vi "Calculate_Release_Flowrates.vi"(3 "Ch names":string[](array[string]), 4 "Units":enum16{"Q l/min", "M_dot Kg/min"}(ring), 5 "Present scan array":dbl[](array[numeric]) format="%.2f") -> (0 "Trace":dbl format="%.2f", 1 "Carrier":dbl format="%.2f", 2 "Scan comments":string)   [LabVIEW 2010]
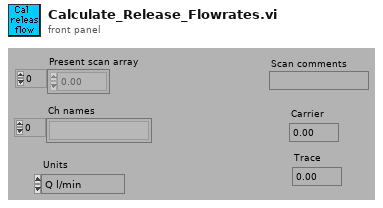
[diagram p1: front panel]
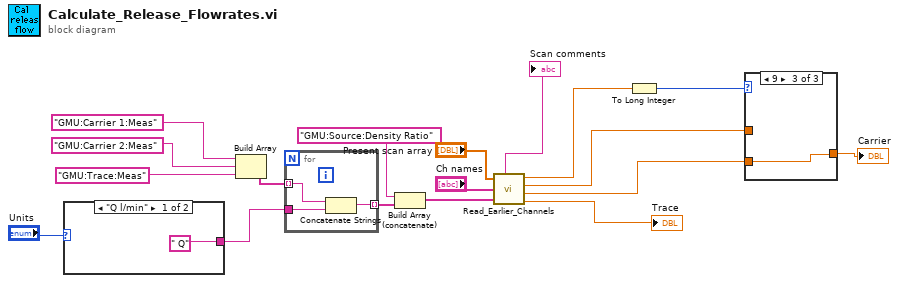
[diagram p0: block diagram]
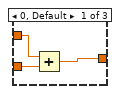
[diagram p2: hidden frame]
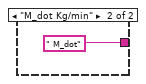
[diagram p4: hidden frame]
diagram:
  n1 = case shown="\"Q l/min\"" "Units" {
    tunnel: [" Q" " M_dot"] -> w17
    frame "Q l/min" {
    }
    frame "M_dot Kg/min" {
    }
  }
  n2 = Build Array("GMU:Carrier 1:Meas", "GMU:Carrier 2:Meas", "GMU:Trace:Meas") -> (w16:string[])
  n3 = for {
    tunnel: w17 -> [w23]
    tunnel: w16 -> [w22] mode=indexing
    tunnel: [w21] -> w9 mode=indexing
    n4 = Concatenate Strings(w22, w23) -> (w21:string)
  }
  n5 = Build Array (concatenate)("GMU:Source:Density Ratio", w9) -> (w10:string[])
  n6 = call "Read_Earlier_Channels.vi"("Present scan array"="Present scan array", "Ch names"="Ch names", "Desired Channels"=w10) -> ("Scan comments"=→"Scan comments":string, "Index 0"=w4:dbl, "Index 1"=w3:dbl, "Index 2"=w2:dbl, "Index 3"=→"Trace":dbl)  [unwired: 1 out]
  n7 = To Long Integer(number=w4) -> (32bit integer=w11:i32)
  n8 = case shown="9" w11 {
    tunnel: w2 -> [w26 _ w28]
    tunnel: w3 -> [w25 w27 _]
    tunnel: [w24 w27 w28] -> w12
    frame 0, Default {
      n9 = Add(x=w25, y=w26) -> (x+y=w24:dbl)
    }
    frame 8 {
    }
    frame 9 {
    }
  }
  "Carrier" <- w12
